vi "ElevatorSim_Pack_Simulation_Params.vi"(8 "SimulateGravity":bool=TRUE, 9 "Measurment StdDev":dbl=0.09, 10 "MaxHeight_Meters":dbl, 11 "MinHeight_Meters":dbl) -> (3 "ElevatorSim_Simulation _Params":T1 {"Measurment StdDev" format="%#_13g"})   [LabVIEW 2019, in "Trajectory_Library.lvlib"]
doc: "Pack simulation parameters used by the Elevator Simulation Execute routine.\n\nInputs:\n - Min Height -- double -- Minimum physical elevator height (meters)\n - Max Height -- double -- Maximum physical elevator height (meters)\n - Pos Sim Std Dev -- double -- Standard deviation for the motor position (meters Default: 0.09)\n - SimulateGravity -- boolean -- Simulate gravity (Default: True)\n\nOutputs:\n - Elevator Sim Simulation -- cluster -- Packed data for Execute function"
uses:
  Trajectory_Library.lvlib
  TypeDef/ELEVATOR_SIM_SIMULATION_PARAMS.ctl
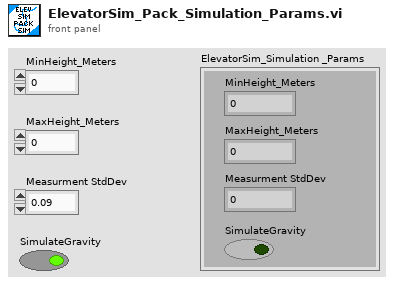
[diagram p1: front panel]
types:
  T1 = typedef "Trajectory_Library.lvlib/ELEVATOR_SIM_SIMULATION_PARAMS.ctl" = cluster{"MinHeight_Meters":dbl, "MaxHeight_Meters":dbl, "Measurment StdDev":dbl, "SimulateGravity":bool}
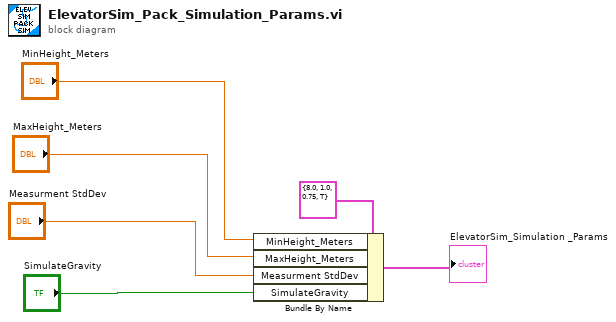
[diagram p0: block diagram]
diagram:
  n1 = Bundle By Name(cluster=T1 {"MinHeight_Meters"=8.0, "MaxHeight_Meters"=1.0, "Measurment StdDev"=0.75, "SimulateGravity"=TRUE} ("SngJntArmSim_Simulation _Params"), "MinHeight_Meters"="MinHeight_Meters", "MaxHeight_Meters"="MaxHeight_Meters", "Measurment StdDev"="Measurment StdDev", "SimulateGravity"="SimulateGravity") -> (→"ElevatorSim_Simulation _Params":T1)
